vi "EnqueueSubVIs.vi"(5 "SubVIs":variant, 6 "error in":errorcluster, 9 "queue":refnum<queue>) -> (0 "error out":errorcluster, 3 "queue out":refnum<queue>)   [LabVIEW 2014, in "Raspberry Pi Compatible Compiler for LabVIEW.lvlib" / "RasPi Compiler.lvclass"]
uses:
  RasPi Compiler.lvclass
  VI Interpreter/Classes/SubVI/SubVI.lvclass
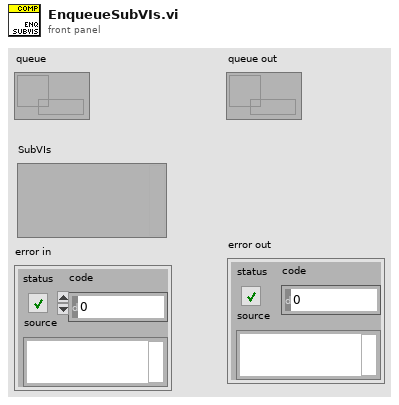
[diagram p1: front panel]
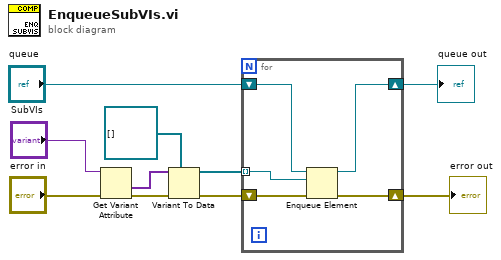
[diagram p0: block diagram]
diagram:
  n1 = Get Variant Attribute(Variant="SubVIs", error in="error in") -> (values=w6:variant[], error out=w8:errorcluster)  [unwired: 2 in, 2 out]
  n2 = Variant To Data(error in=w8, type=refnum<class "SubVI.lvclass">[] [], Variant=w6) -> (data=w10:refnum<class "SubVI.lvclass">[], error out=w4:errorcluster)
  n3 = for {
    shift-right: [w12] -> w2
    shift-left: "queue" -> [w14]
    shift-right: [w11] -> w1
    shift-left: w4 -> [w15]
    tunnel: w10 -> [w13] mode=indexing
    n4 = Enqueue Element(queue=w14, element=w13, error in (no error)=w15) -> (queue out=w12:refnum<queue>, error out=w11:errorcluster)  [unwired: 1 in, 1 out]
  }
  "queue out" <- w2
  "error out" <- w1
